vi "Funct TIFF export-Core.vi"(8 "error in (no error)":errorcluster, 9 "Experiment Header string":refnum<vi>, 10 "ProgressBar":refnum<k24>, 11 "Info indicators only (F)":bool) -> ()   [LabVIEW 2020]
uses:
  System.Windows.Forms
  Globals/gl_funct TIFF export globals.vi
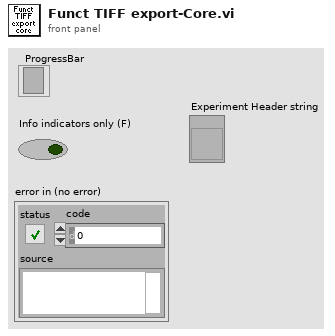
[diagram p1: front panel]
types:
  T1 = typedef "Funct TIFF exporter ctrl refs.ctl" = cluster{"This VI":refnum<vi>, "Current Experiment":refnum<vi>, "Imaging protocol":refnum<vi>, "Predominant ROI type":refnum<vi>, "Patches in Experiment":refnum<vi>, "Folder Path":refnum<vi>, "Export":refnum<vi>, "Trial number":refnum<vi>, "Output TIFF type":refnum<vi>}
  T2 = typedef "ROI ID Enum.ctl" = enum16{"Point", "MiniScan", "Comp. MiniScan", "Rectangle", "Comp. volume", "Arb. plane point", "None"}
  T3 = typedef "Imaging Protocols enum.ctl" = enum16{"AOL Z-Stack", "Motor Z Stack", "Functional Acquisition", "Single Plane Acquisition", "Volume Acquisition", "Live Imaging", "Live Plane Imaging", "Live Volume Imaging"}
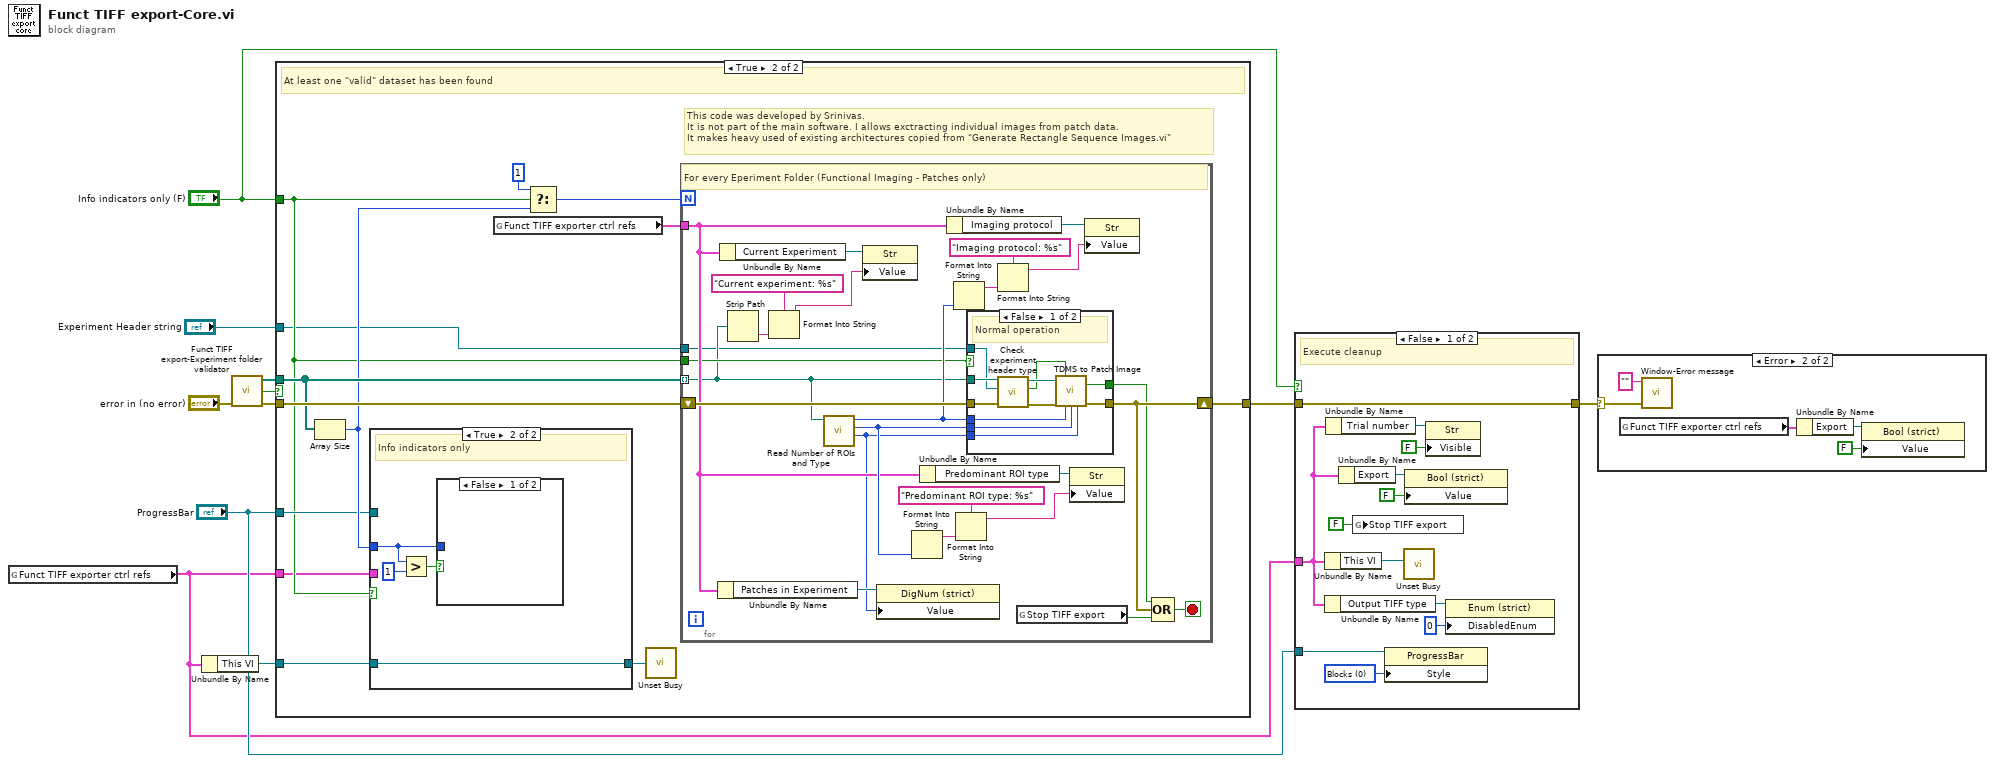
[diagram p0: block diagram]
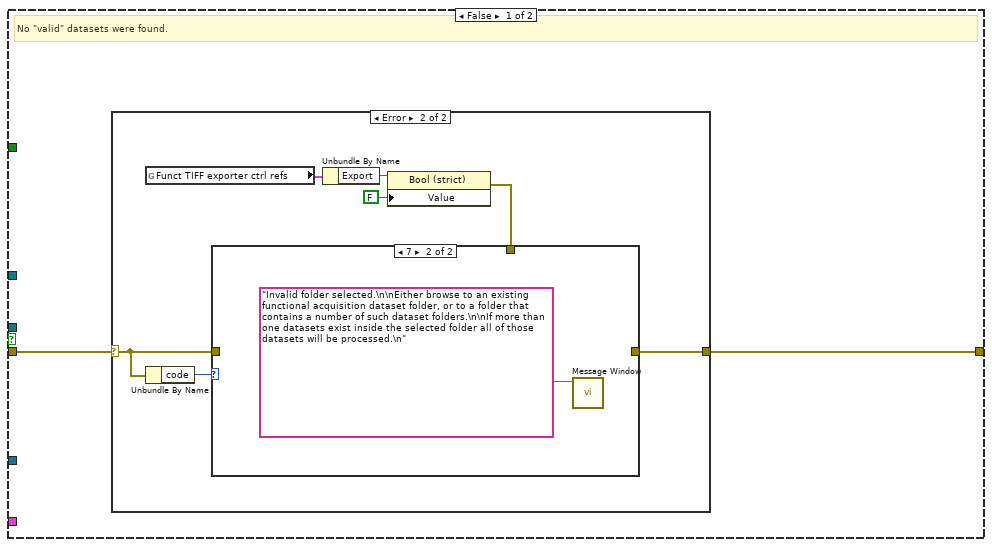
[diagram p4: hidden frame]
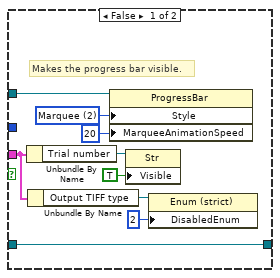
[diagram p7: hidden frame]
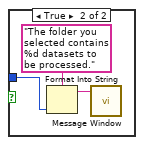
[diagram p8: hidden frame]
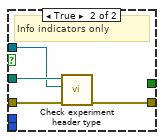
[diagram p9: hidden frame]
diagram:
  n1 = global read "gl_funct TIFF export globals.vi" "Funct TIFF exporter ctrl refs"() -> (w4:T1)
  n2 = Unbundle By Name(w4) -> ("This VI"=w7:refnum<vi>)
  n3 = call "Funct TIFF export-Experiment folder validator.vi"("error in (no error)"="error in (no error)") -> ("error out"=w11:errorcluster, "Valid experiment folders found"=w8:bool, "Filtered Array out"=w9:path[])  [unwired: 8 in]
  n4 = case shown="True" w8 {
    tunnel: w11 -> [w13 w36]
    tunnel: "Info indicators only (F)" -> [_ w26]
    tunnel: [w12 w33] -> w3
    tunnel: w9 -> [_ w31]
    tunnel: w7 -> [_ w29]
    tunnel: "ProgressBar" -> [_ w27]
    tunnel: w4 -> [_ w25]
    tunnel: "Experiment Header string" -> [_ w24]
    frame False {
      # "No \"valid\" datasets were found."
      n5 = case shown="Error" w13 {
        selector: w13 -> [w14 w20]
        tunnel: [w14 w19] -> w12
        frame No Error {
        }
        frame Error {
          n6 = global read "gl_funct TIFF export globals.vi" "Funct TIFF exporter ctrl refs"() -> (w18:T1)
          n7 = Unbundle By Name(w20) -> ("code"=w21:i32)
          n8 = Unbundle By Name(w18) -> ("Export"=w17:refnum<vi>)
          n9 = property class="Bool (strict)"(reference=w17, "Value"=FALSE) -> (error out=w15:errorcluster)  [unwired: 1 in, 1 out]
          n10 = case shown="7" w21 {
            tunnel: [w22 _] -> w19
            tunnel: w20 -> [w22 _]
            tunnel: w15 -> [_ _]
            frame 0, Default {
            }
            frame 7 {
              n11 = call "Message Window.vi"("Message string"="Invalid folder selected.\n\nEither browse to an existing functional acquisition dataset folder, or to a folder that contains a number of such dataset folders.\n\nIf more than one datasets exist inside the selected folder all of those datasets will be processed.\n") -> ()  [unwired: 10 in, 1 out]
            }
          }
        }
      }
    }
    frame True {
      # "This code was developed by Srinivas.\nIt is not part of the main software. I allows exctracting individual images from patch data.\nIt makes heavy used of existing architectures copied from \"Generate Rectangle Sequence Images.vi\""
      # "At least one \"valid\" dataset has been found"
      n12 = Array Size(array=w31) -> (size(s)=w30:i32)
      n13 = case shown="True" w26 {
        tunnel: w30 -> [_ w47]
        tunnel: [w45 w46] -> w28
        tunnel: w29 -> [w45 w46]
        tunnel: w27 -> [w44 _]
        tunnel: w25 -> [w38 _]
        frame False {
          w43 = 2 items=["Blocks", "Continuous", "Marquee"] ("Style")
          # "Makes the progress bar visible."
          n14 = Unbundle By Name(w38) -> ("Trial number"=w41:refnum<vi>)
          n15 = Unbundle By Name(w38) -> ("Output TIFF type"=w39:refnum<vi>)
          n16 = property class="ProgressBar"(reference=w44, "Style"=w43, "MarqueeAnimationSpeed"=20) -> ()  [unwired: 1 in, 2 out]
          n17 = property class="Str"(reference=w41, "Visible"=TRUE) -> ()  [unwired: 1 in, 2 out]
          n18 = property class="Enum (strict)"(reference=w39, "DisabledEnum"=2) -> ()  [unwired: 1 in, 2 out]
        }
        frame True {
          # "Info indicators only"
          n19 = Greater?(x=w47, y=1) -> (0:w48:bool)
          n20 = case shown="False" w48 {
            tunnel: w47 -> [_ w52]
            frame False {
            }
            frame True {
              n21 = Format Into String(format string="The folder you selected contains %d datasets to be processed.", w52) -> (resulting string=w50:string)  [unwired: 2 in, 1 out]
              n22 = call "Message Window.vi"("Message string"=w50) -> ()  [unwired: 10 in, 1 out]
            }
          }
        }
      }
      n23 = global read "gl_funct TIFF export globals.vi" "Funct TIFF exporter ctrl refs"() -> (w32:T1)
      n24 = Select(t=1, s=w26, f=w30) -> (s? t:f=w34:i32)
      n25 = call <vilib>:"Unset Busy.vi"("VI reference (current VI)"=w28) -> ()  [unwired: 10 in, 1 out]
      n26 = for {
        N: w34 -> [_]
        tunnel: w31 -> [w56] mode=indexing
        tunnel: w32 -> [w62]
        tunnel: w26 -> [w60]
        shift-right: [w57] -> w33
        shift-left: w36 -> [w77]
        tunnel: w24 -> [w53]
        stop <- w59 stop-if-true
        # "For every Eperiment Folder (Functional Imaging - Patches only)"
        n27 = Unbundle By Name(w62) -> ("Patches in Experiment"=w63:refnum<vi>)
        n28 = Unbundle By Name(w62) -> ("Current Experiment"=w69:refnum<vi>)
        n29 = Strip Path(path=w56) -> (name=w55:string)  [unwired: 1 out]
        n30 = Format Into String(format string="Current experiment: %s", w55) -> (resulting string=w68:string)  [unwired: 2 in, 1 out]
        n31 = call "Read Number of ROIs and Type.vi"("Experimental Folder"=w56) -> ("Patches in Experiment"=w61:i32, "Predominant ROI type"=w70:T2, "Imaging Protocol"=w75:T3)  [unwired: 8 in]
        n32 = property class="Str"(reference=w69, "Value"=w68) -> ()  [unwired: 1 in, 2 out]
        n33 = property class="DigNum (strict)"(reference=w63, "Value"=w61) -> ()  [unwired: 1 in, 2 out]
        n34 = Format Into String(w70) -> (resulting string=w72:string)  [unwired: 3 in, 1 out]
        n35 = Unbundle By Name(w62) -> ("Predominant ROI type"=w65:refnum<vi>)
        n36 = Unbundle By Name(w62) -> ("Imaging protocol"=w67:refnum<vi>)
        n37 = Format Into String(w75) -> (resulting string=w74:string)  [unwired: 3 in, 1 out]
        n38 = Format Into String(format string="Predominant ROI type: %s", w72) -> (resulting string=w64:string)  [unwired: 2 in, 1 out]
        n39 = case shown="False" w60 {
          tunnel: [w88 w90] -> w57
          tunnel: w77 -> [w83 w91]
          tunnel: w75 -> [w87 _]
          tunnel: w70 -> [w86 _]
          tunnel: w61 -> [w85 _]
          tunnel: w56 -> [w81 w92]
          tunnel: [w84 _] -> w54
          tunnel: w53 -> [w78 w89]
          frame False {
            # "Normal operation"
            n40 = call "Check experiment header type.vi"("error in (no error)"=w83, "Experiment Header string"=w78, "Path"=w81) -> ("error out"=w82:errorcluster, "Old format ?"=w79:bool, "Path- out"=w80:path)  [unwired: 6 in]
            n41 = call "TDMS to Patch Image.vi"("Experiment Path"=w80, "Old Version"=w79, "error in (no error)"=w82, "Imaging Protocol"=w87, "Predominant ROI type"=w86, "No of Patches in Experiment"=w85) -> ("Cancelled"=w84:bool, "error out"=w88:errorcluster)  [unwired: 6 in, 2 out]
          }
          frame True {
            # "Info indicators only"
            n42 = call "Check experiment header type.vi"("error in (no error)"=w91, "Experiment Header string"=w89, "Path"=w92) -> ("error out"=w90:errorcluster)  [unwired: 6 in, 2 out]
          }
        }
        n43 = Format Into String(format string="Imaging protocol: %s", w74) -> (resulting string=w66:string)  [unwired: 2 in, 1 out]
        n44 = global read "gl_funct TIFF export globals.vi" "Stop TIFF export"() -> (w58:bool)
        n45 = property class="Str"(reference=w65, "Value"=w64) -> ()  [unwired: 1 in, 2 out]
        n46 = property class="Str"(reference=w67, "Value"=w66) -> ()  [unwired: 1 in, 2 out]
        n47 = Compound Arithmetic op=OR(w54, w57, w58) -> (w59:bool)
      }
    }
  }
  n48 = case shown="False" "Info indicators only (F)" {
    tunnel: "ProgressBar" -> [w102 _]
    tunnel: w4 -> [w93 _]
    tunnel: w3 -> [w96 w105]
    tunnel: [w96 w105] -> w2
    frame False {
      w103 = 0 items=["Blocks", "Continuous", "Marquee"] ("Style")
      # "Execute cleanup"
      n49 = Unbundle By Name(w93) -> ("This VI"=w101:refnum<vi>)
      n50 = Unbundle By Name(w93) -> ("Output TIFF type"=w95:refnum<vi>)
      n51 = Unbundle By Name(w93) -> ("Trial number"=w97:refnum<vi>)
      n52 = Unbundle By Name(w93) -> ("Export"=w100:refnum<vi>)
      n53 = global write "gl_funct TIFF export globals.vi" "Stop TIFF export"(FALSE ("Stop TIFF export")) -> ()
      n54 = property class="ProgressBar"(reference=w102, "Style"=w103) -> ()  [unwired: 1 in, 2 out]
      n55 = call <vilib>:"Unset Busy.vi"("VI reference (current VI)"=w101) -> ()  [unwired: 10 in, 1 out]
      n56 = property class="Bool (strict)"(reference=w100, "Value"=FALSE ("Export")) -> ()  [unwired: 1 in, 2 out]
      n57 = property class="Str"(reference=w97, "Visible"=FALSE) -> ()  [unwired: 1 in, 2 out]
      n58 = property class="Enum (strict)"(reference=w95, "DisabledEnum"=0) -> ()  [unwired: 1 in, 2 out]
    }
    frame True {
      # "Info indicators only"
    }
  }
  n59 = case shown="Error" w2 {
    selector: w2 -> [_ w110]
    frame No Error {
    }
    frame Error {
      n60 = global read "gl_funct TIFF export globals.vi" "Funct TIFF exporter ctrl refs"() -> (w106:T1)
      n61 = call "Window-Error message.vi"("error in (no error)"=w110, "Message"="") -> ()  [unwired: 9 in, 1 out]
      n62 = Unbundle By Name(w106) -> ("Export"=w107:refnum<vi>)
      n63 = property class="Bool (strict)"(reference=w107, "Value"=FALSE) -> ()  [unwired: 1 in, 2 out]
    }
  }
